vi "set current.vi"(8 "error in (no error)":errorcluster, 10 "Current [A]":dbl, 11 "BK 9202B in":refnum<class "BK 9202B.lvclass">) -> (0 "error out":errorcluster, 3 "BK 9202B out":refnum<class "BK 9202B.lvclass">)   [LabVIEW 2025, in "Power Supply.lvlib" / "BK 9202B.lvclass"]
uses:
  BK 9202B.lvclass
  BK 9202B.lvclass/BK 9202B.ctl
  generic-power-supply/generic-power-supply.lvclass
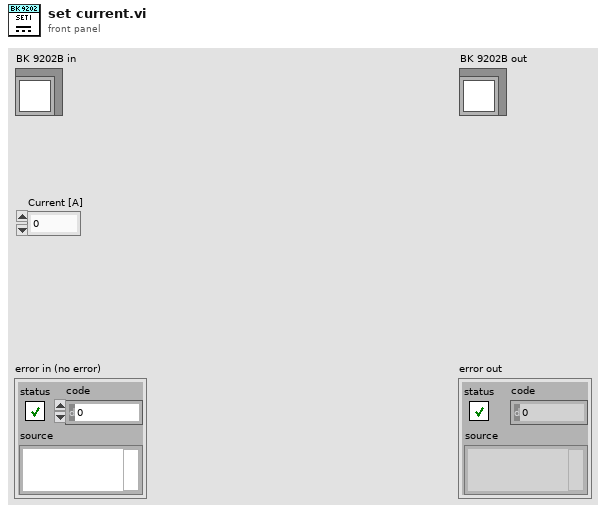
[diagram p1: front panel]
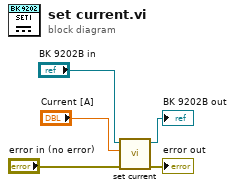
[diagram p0: block diagram]
diagram:
  n1 = call-parent "set current.vi"("error in (no error)"="error in (no error)", "Current [A]"="Current [A]", "generic-power-supply in"="BK 9202B in") -> ("error out"=→"error out":errorcluster, "generic-power-supply out"=→"BK 9202B out":refnum<class "BK 9202B.lvclass">)  [unwired: 7 in]
